vi "Load YAML Configuration.vi"(8 "Error In":errorcluster, 10 "YAML Config File Path":string) -> (0 "Error Out":errorcluster, 3 "YAML Handle Out":u64)   [LabVIEW 2019, in "YAML Config Reader.lvlib"]
uses:
  YAML Config Reader.lvlib
  target/debug/rust_labview_yaml.dll
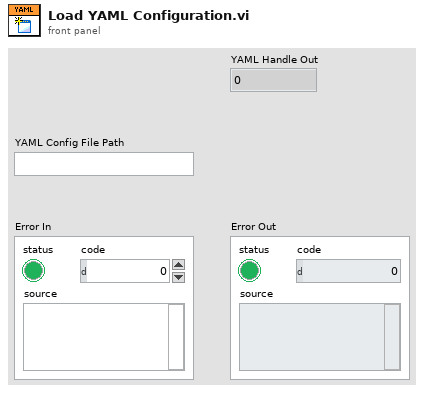
[diagram p1: front panel]
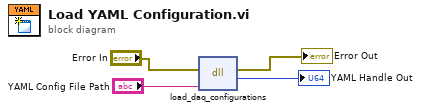
[diagram p0: block diagram]
diagram:
  n1 = dll-call lib="C:/dev/rust_labview_yaml/target/debug/rust_labview_yaml.dll" fn="load_daq_configurations"(error in="Error In", "filepath"="YAML Config File Path") -> (error out=→"Error Out":errorcluster, "return type"=→"YAML Handle Out":u64)  [unwired: 3 in, 1 out]
